vi "Counter.vi"   [LabVIEW 2014]
uses:
  ElevatorStates.ctl
  Global Data!!!.vi
types:
  T1 = typedef "ElevatorStates.ctl" = enum16{"DropSequence", "Reset", "Drop1Stage", "2StageEngage", "Lift1Stage", "1StageEngage", "Rest", "InterruptedLift", "Manual", "Auto2Man", "Initialize", "FeederMode"}
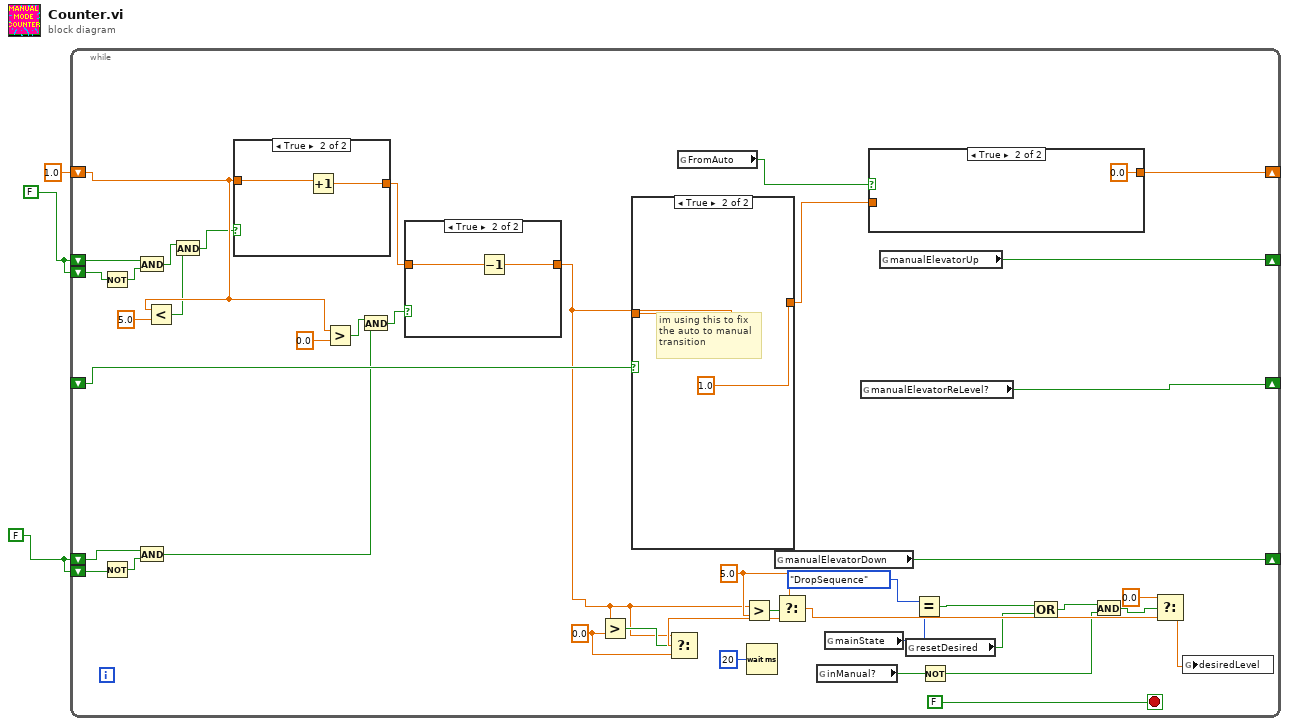
[diagram p0: block diagram]
diagram:
  w1 = FALSE ("Value to be Counted")
  w3 = FALSE ("Value to be Counted")
  n1 = while {
    shift-right: [w38] -> _
    shift-left: w3 -> [w43]
    shift-left: w3 -> [w45]
    shift-right: [w4] -> _
    shift-left: 1.0 -> [w25]
    shift-right: [w37] -> _
    shift-left: w1 -> [w40]
    shift-left: w1 -> [w41]
    shift-right: [w30] -> _
    shift-left: _ -> [w35]
    stop <- FALSE stop-if-true
    w31 = 0.0 ("y")
    w29 = 5.0 ("upper limit")
    n2 = Not(x=w45) -> (.not. x?=w44:bool)
    n3 = Not(x=w41) -> (.not. x?=w42:bool)
    n4 = And(x=w43, y=w44) -> (x .and. y?=w23:bool)
    n5 = And(x=w40, y=w42) -> (x .and. y?=w19:bool)
    n6 = Less?(x=w25, y=5.0) -> (x < y?=w22:bool)
    n7 = And(x=w23, y=w22) -> (x .and. y?=w21:bool)
    n8 = case shown="True" w21 {
      tunnel: w25 -> [w53 w55]
      tunnel: [w53 w54] -> w28
      frame False {
      }
      frame True {
        n9 = Increment(x=w55) -> (x+1=w54:dbl)
      }
    }
    n10 = Greater?(x=w25, y=0.0) -> (0:w20:bool)
    n11 = And(x=w20, y=w19) -> (x .and. y?=w18:bool)
    n12 = case shown="True" w18 {
      tunnel: [w50 w52] -> w27
      tunnel: w28 -> [w50 w51]
      frame False {
      }
      frame True {
        n13 = Decrement(x=w51) -> (x-1=w52:dbl)
      }
    }
    n14 = Greater?(x=w27, y=w31) -> (0:w33:bool)
    n15 = case shown="True" w35 {
      tunnel: w27 -> [w48 _]
      tunnel: [w48 1.0] -> w5
      frame False {
      }
      frame True {
        # "im using this to fix\nthe auto to manual\ntransition"
      }
    }
    n16 = Select(t=w27, s=w33, f=w31) -> (s? t:f=w34:dbl)
    n17 = global read "Global Data!!!.vi" "FromAuto"() -> (w6:bool)
    n18 = Greater?(x=w27, y=w29) -> (0:w32:bool)
    n19 = Wait (ms)(milliseconds to wait=u32 20) -> ()  [unwired: 1 out]
    n20 = global read "Global Data!!!.vi" "manualElevatorDown"() -> (w37:bool)
    n21 = Select(t=w29, s=w32, f=w34) -> (s? t:f=w17:dbl)
    n22 = global read "Global Data!!!.vi" "inManual?"() -> (w12:bool)
    n23 = global read "Global Data!!!.vi" "mainState"() -> (w14:i8)
    n24 = global read "Global Data!!!.vi" "manualElevatorReLevel?"() -> (w30:bool)
    n25 = case shown="True" w6 {
      tunnel: w5 -> [w46 _]
      tunnel: [w46 0.0] -> w4
      frame False {
      }
      frame True {
      }
    }
    n26 = global read "Global Data!!!.vi" "manualElevatorUp"() -> (w38:bool)
    n27 = global read "Global Data!!!.vi" "resetDesired"() -> (w8:bool)
    n28 = Equal?(x=ElevatorStates."DropSequence" ("Enum"), y=w14) -> (x = y?=w10:bool)
    n29 = Not(x=w12) -> (.not. x?=w11:bool)
    n30 = Compound Arithmetic op=OR(w10, w8) -> (w9:bool)
    n31 = And(x=w9, y=w11) -> (x .and. y?=w13:bool)
    n32 = Select(t=0.0, s=w13, f=w17) -> (s? t:f=w7:dbl)
    n33 = global write "Global Data!!!.vi" "desiredLevel"(w7) -> ()
  }
